vi "Replace Wheels.vi"(5 "x positions":dbl[](array[numeric]), 6 "frame angles (rad)":dbl[](array[numeric]), 7 "y positions":dbl[](array[numeric]), 8 "error in (no error)":errorcluster, 9 "wheels":refnum<class "NI_Robotics_Wheel.lvclass">[](array[class]), 10 "wheel indexes":i32[](array[numeric]), 11 "steering frame in":refnum<class "NI_Robotics_Steering Frame.lvclass">) -> (0 "error out":errorcluster, 1 "found?":bool[](array[boolean]), 3 "steering frame out":refnum<class "NI_Robotics_Steering Frame.lvclass">)   [LabVIEW 2017, in "NI_Robotics_Steering Frame.lvclass"]
uses:
  <vilib>/robotics/Steering/Steering Frame/NI_Robotics_Steering Frame.lvclass
  <vilib>/robotics/Steering/Wheel/NI_Robotics_Wheel.lvclass
  <vilib>/robotics/Steering/Steering Frame/NI_Robotics_Steering Frame.lvclass/NI_Robotics_Steering Frame.ctl
  <vilib>/robotics/Steering/Wheel/NI_Robotics_Wheel.lvclass/NI_Robotics_Wheel.ctl
  <vilib>/Analysis/coordinate.llb/Wrap Angle (scalar).vi
  <vilib>/Analysis/NI_AAL_Angle.lvlib
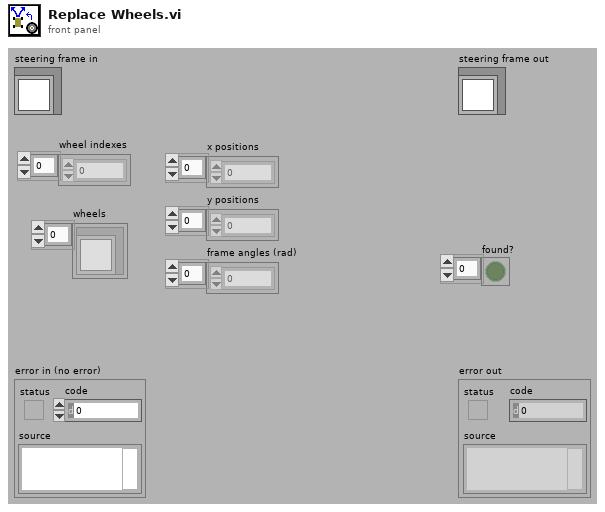
[diagram p1: front panel]
types:
  T1 = typedef "NI_Robotics_Wheel.lvclass/Wheel State.ctl" = cluster{"wheel name":string, "forward angular velocity":dbl, "caster angular velocity":dbl, "caster wheel angle (rad)":dbl, "steering angle (rad)":dbl}
  T2 = typedef "NI_Robotics_Steering Frame.lvclass/Wheel Orientation.ctl" = cluster{"wheel":refnum<class "NI_Robotics_Wheel.lvclass">, "x position":dbl, "y position":dbl, "frame angle (rad)":dbl}
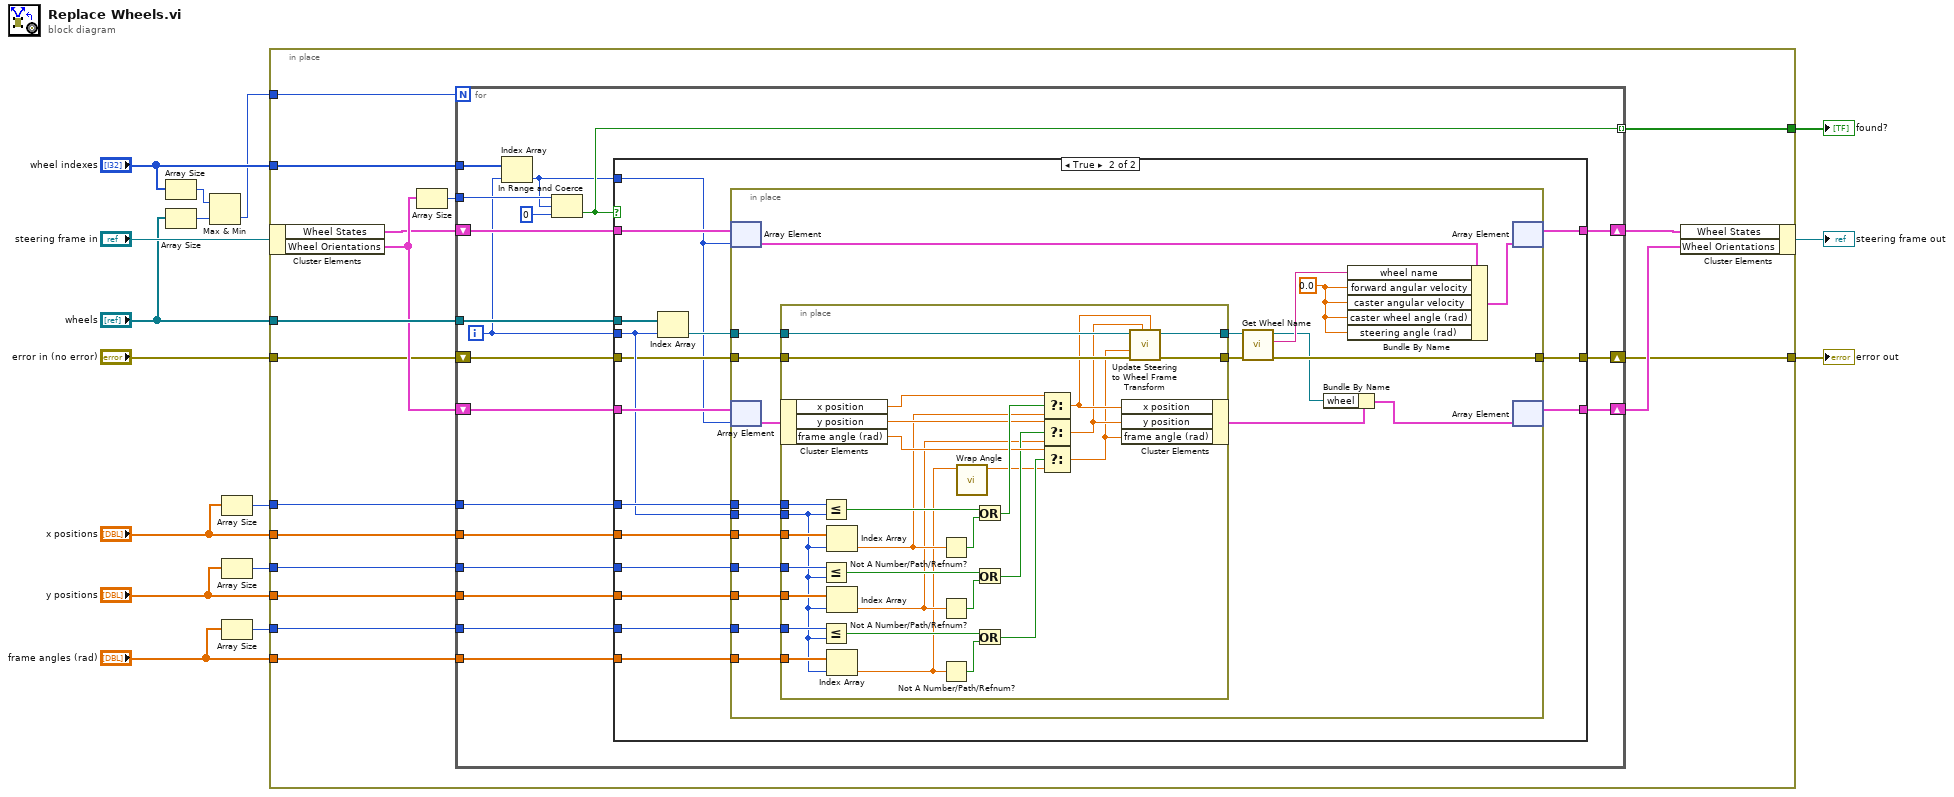
[diagram p0: block diagram]
diagram:
  n1 = Array Size(array="wheel indexes") -> (size(s)=w9:i32)
  n2 = Array Size(array="wheels") -> (size(s)=w10:i32)
  n3 = Max & Min(x=w9, y=w10) -> (min(x,y)=w7:i32)  [unwired: 1 out]
  n4 = Array Size(array="x positions") -> (size(s)=w5:i32)
  n5 = Array Size(array="y positions") -> (size(s)=w2:i32)
  n6 = Array Size(array="frame angles (rad)") -> (size(s)=w1:i32)
  n7 = in-place {
    in-place-border: "wheels" -> [w32]
    in-place-border: "wheel indexes" -> [w20]
    in-place-border: [w29] -> w12
    in-place-border: "x positions" -> [w28]
    in-place-border: "y positions" -> [w27]
    in-place-border: "frame angles (rad)" -> [w26]
    in-place-border: "error in (no error)" -> [w25]
    in-place-border: [w24] -> w13
    in-place-border: w7 -> [w21]
    in-place-border: w5 -> [w19]
    in-place-border: w2 -> [w18]
    in-place-border: w1 -> [w17]
    n8 = in-place-cluster #1("steering frame in") -> ("Wheel States"=w23:T1[], "Wheel Orientations"=w31:T2[])
    n9 = Array Size(array=w31) -> (size(s)=w30:i32)
    n10 = for {
      N: w21 -> [_]
      shift-right: [w51] -> w33
      shift-left: w31 -> [w52]
      tunnel: w32 -> [w43]
      tunnel: w30 -> [w47]
      tunnel: [w48] -> w29 mode=indexing
      tunnel: w28 -> [w50]
      tunnel: w27 -> [w35]
      tunnel: w26 -> [w49]
      shift-right: [w41] -> w24
      shift-left: w25 -> [w42]
      shift-right: [w44] -> w22
      shift-left: w23 -> [w45]
      tunnel: w20 -> [w40]
      tunnel: w19 -> [w37]
      tunnel: w18 -> [w36]
      tunnel: w17 -> [w34]
      i -> [w38]
      n11 = Index Array(array=w40, index=w38) -> (element=w39:i32)
      n12 = In Range and Coerce(upper limit=w47, x=w39, lower limit=0) -> (In Range?=w48:bool)  [unwired: 1 out]
      n13 = case shown="True" w48 {
        tunnel: w52 -> [w55 w69]
        tunnel: w43 -> [_ w70]
        tunnel: [w55 w68] -> w51
        tunnel: w39 -> [_ w56]
        tunnel: w50 -> [_ w67]
        tunnel: w49 -> [_ w61]
        tunnel: w45 -> [w54 w58]
        tunnel: [w54 w57] -> w44
        tunnel: w42 -> [w53 w59]
        tunnel: [w53 w71] -> w41
        tunnel: w38 -> [_ w65]
        tunnel: w37 -> [_ w66]
        tunnel: w36 -> [_ w64]
        tunnel: w35 -> [_ w63]
        tunnel: w34 -> [_ w62]
        frame False {
          # "Index is out of range.  Do nothing."
        }
        frame True {
          n14 = Index Array(array=w70, index=w65) -> (element=w60:refnum<class "NI_Robotics_Wheel.lvclass">)
          n15 = in-place {
            in-place-border: w67 -> [w90]
            in-place-border: w66 -> [w89]
            in-place-border: w65 -> [w88]
            in-place-border: w64 -> [w87]
            in-place-border: w63 -> [w86]
            in-place-border: w62 -> [w85]
            in-place-border: w61 -> [w84]
            in-place-border: w60 -> [w83]
            in-place-border: [w76] -> w71
            in-place-border: w59 -> [w82]
            w81 = 0.0 ("forward angular velocity")
            n16 = in-place-array #2(w58, w56) -> (w80:T1)
            n17 = in-place-array #3(w69, w56) -> (w91:T2)
            n18 = in-place {
              in-place-border: w90 -> [w121]
              in-place-border: w89 -> [w120]
              in-place-border: w88 -> [w104]
              in-place-border: w87 -> [w113]
              in-place-border: w86 -> [w112]
              in-place-border: w85 -> [w106]
              in-place-border: w84 -> [w105]
              in-place-border: w83 -> [w100]
              in-place-border: [w99] -> w78
              in-place-border: [w98] -> w77
              in-place-border: w82 -> [w97]
              n19 = in-place-cluster #4(w91) -> ("x position"=w116:dbl, "y position"=w115:dbl, "frame angle (rad)"=w114:dbl)
              n20 = Less Or Equal?(x=w120, y=w104) -> (x <= y?=w118:bool)
              n21 = Less Or Equal?(x=w113, y=w104) -> (x <= y?=w109:bool)
              n22 = Less Or Equal?(x=w106, y=w104) -> (x <= y?=w102:bool)
              n23 = Index Array(array=w121, index=w104) -> (element=w111:dbl)
              n24 = Index Array(array=w112, index=w104) -> (element=w107:dbl)
              n25 = Index Array(array=w105, index=w104) -> (element=w93:dbl)
              n26 = Not A Number/Path/Refnum?(number/path/refnum=w111) -> (NaN/Path/Refnum?=w119:bool)
              n27 = Not A Number/Path/Refnum?(number/path/refnum=w107) -> (NaN/Path/Refnum?=w110:bool)
              n28 = Not A Number/Path/Refnum?(number/path/refnum=w93) -> (NaN/Path/Refnum?=w103:bool)
              n29 = call-poly <vilib>:"Wrap Angle.vi"("angle in"=w93) -> ("angle out"=w92:dbl)  [unwired: 9 in, 1 out]
              n30 = Or(x=w118, y=w119) -> (x .or. y?=w117:bool)
              n31 = Or(x=w109, y=w110) -> (x .or. y?=w108:bool)
              n32 = Or(x=w102, y=w103) -> (x .or. y?=w101:bool)
              n33 = Select(t=w116, s=w117, f=w111) -> (s? t:f=w96:dbl)
              n34 = Select(t=w115, s=w108, f=w107) -> (s? t:f=w95:dbl)
              n35 = Select(t=w114, s=w101, f=w92) -> (s? t:f=w94:dbl)
              n36 = in-place-cluster #4("x position"=w96, "y position"=w95, "frame angle (rad)"=w94) -> (w74:T2)
              n37 = call <vilib>:"Update Steering to Wheel Frame Transform.vi"("x wheel position"=w96, "y wheel position"=w95, "error in (no error)"=w97, "wheel frame angle (rad)"=w94, "wheel in"=w100) -> ("error out"=w98:errorcluster, "wheel out"=w99:refnum<class "NI_Robotics_Wheel.lvclass">)  [unwired: 5 in]
            }
            n38 = call <vilib>:"Get Wheel Name.vi"("error in (no error)"=w77, "wheel in"=w78) -> ("error out"=w76:errorcluster, "wheel name"=w75:string, "wheel out"=w72:refnum<class "NI_Robotics_Wheel.lvclass">)  [unwired: 7 in]
            n39 = Bundle By Name(cluster=w74, "wheel"=w72) -> (w73:T2)
            n40 = Bundle By Name(cluster=w80, "wheel name"=w75, "forward angular velocity"=w81, "caster angular velocity"=w81, "caster wheel angle (rad)"=w81, "steering angle (rad)"=w81) -> (w79:T1)
            n41 = in-place-array #2(w79) -> (w57:T1[])  [unwired: 1 out]
            n42 = in-place-array #3(w73) -> (w68:T2[])  [unwired: 1 out]
          }
        }
      }
    }
    n43 = in-place-cluster #1("Wheel States"=w22, "Wheel Orientations"=w33) -> (→"steering frame out":refnum<class "NI_Robotics_Steering Frame.lvclass">)
  }
  "error out" <- w13
  "found?" <- w12
